vi "Setup subWorker - AcquireWorker.vi"(8 "error in":errorcluster, 11 "ChartView Worker in":refnum<class "ChartView Worker.lvclass">) -> (0 "error out":errorcluster, 3 "ChartView Worker out":refnum<class "ChartView Worker.lvclass">)   [LabVIEW 2018, in "ChartView Worker.lvclass"]
doc: "<b>Note: Do not change the code in this VI!</b>\nThis VI performs a setup of all the statically-linked subWorkers that belong to the Worker that calls this VI. This VI is created automatically by the 'Create/Add Worker' tool and must be called <b>before</b> any statically linked subWorkers are called."
uses:
  ChartView Worker.lvclass
  ChartView Worker.lvclass/ChartView Worker.ctl
  Acquire Worker/DataAcquire Worker.lvclass
  D:/Program Files (x86)/National Instruments/LabVIEW 2018/vi.lib/addons/_Workers/Library/Classes/Worker/Worker.lvclass
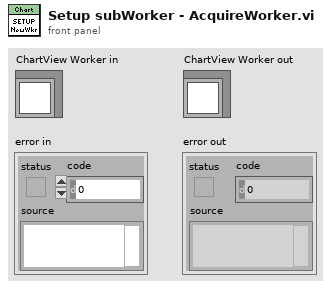
[diagram p1: front panel]
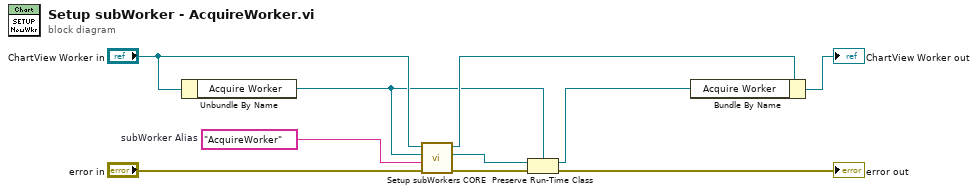
[diagram p0: block diagram]
diagram:
  w6 = "AcquireWorker"  # subWorker Alias
  n1 = Unbundle By Name("ChartView Worker in") -> ("Acquire Worker"=w3:refnum<class "DataAcquire Worker.lvclass">)
  n2 = call-dynamic "Setup subWorkers CORE.vi"("error in"="error in", "subWorker Alias"=w6, "subWorker"=w3, "Worker"="ChartView Worker in") -> ("error out"=w5:errorcluster, "subWorker out"=w1:refnum<class "Worker.lvclass">, "Worker out"=w8:refnum<class "ChartView Worker.lvclass">)  [unwired: 5 in]
  n3 = Preserve Run-Time Class(object in=w1, error in=w5, 2:w3) -> (object out=w2:refnum<class "DataAcquire Worker.lvclass">, error out=→"error out":errorcluster)
  n4 = Bundle By Name(cluster=w8, "Acquire Worker"=w2) -> (→"ChartView Worker out":refnum<class "ChartView Worker.lvclass">)
